vi "Control Mode.vi"(8 "Error In":errorcluster, 10 "Control Mode":bool, 11 "KIT-QVA in":refnum<class "KIT-QVA.lvclass">) -> (0 "Error Out":errorcluster, 3 "KIT-QVA out":refnum<class "KIT-QVA.lvclass">)   [LabVIEW 2014, in "KIT-QVA.lvlib" / "KIT-QVA.lvclass"]
doc: "Start or stop control mode."
uses:
  KIT-QVA.lvclass
  KIT-QVA.lvclass/KIT-QVA.ctl
  instr.lib/KIT-QV/KIT QV.lvlib
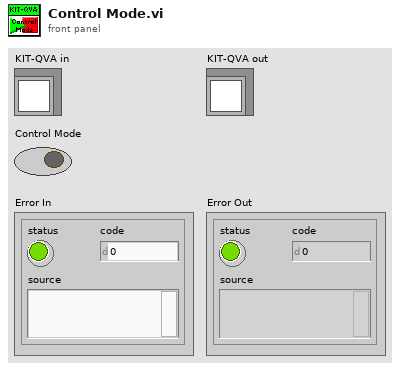
[diagram p1: front panel]
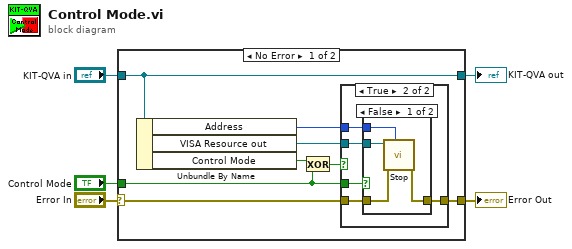
[diagram p0: block diagram]
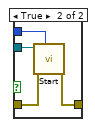
[diagram p3: hidden frame]
diagram:
  n1 = case shown="No Error" "Error In" {
    selector: "Error In" -> [w8 w29]
    tunnel: [w6 w29] -> w4
    tunnel: [w13 w28] -> w2
    tunnel: "KIT-QVA in" -> [w13 w28]
    tunnel: "Control Mode" -> [w7 _]
    frame No Error {
      n2 = Unbundle By Name(w13) -> ("Address"=w11:u16, "VISA Resource out"=w12:refnum<visa-resource-name>, "Control Mode"=w10:bool)
      n3 = Exclusive Or(1:w7, 2:w10) -> (0:w9:bool)
      n4 = case shown="True" w9 {
        tunnel: w12 -> [_ w19]
        tunnel: w11 -> [_ w18]
        tunnel: w8 -> [w14 w17]
        tunnel: w7 -> [_ w16]
        tunnel: [w14 w15] -> w6
        frame False {
        }
        frame True {
          n5 = case shown="False" w16 {
            tunnel: w19 -> [w23 w27]
            tunnel: w18 -> [w22 w26]
            tunnel: w17 -> [w21 w25]
            tunnel: [w20 w24] -> w15
            frame False {
              n6 = call "Stop.vi"("Address"=w22, "Error In"=w21, "VISA Resource in"=w23) -> ("Error Out"=w20:errorcluster)  [unwired: 7 in, 1 out]
            }
            frame True {
              n7 = call "Start.vi"("Address"=w26, "Error In"=w25, "VISA Resource in"=w27) -> ("Error Out"=w24:errorcluster)  [unwired: 7 in, 1 out]
            }
          }
        }
      }
    }
    frame Error {
    }
  }
  "Error Out" <- w4
  "KIT-QVA out" <- w2
